vi "cast_meta_idx_toINT.vi"(11 "2D Data Out":sgl[][](array[numeric])) -> (3 "output array":sgl[][](array[numeric]))   [LabVIEW 2017]
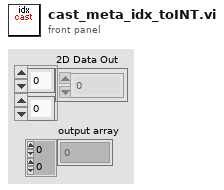
[diagram p1: front panel]
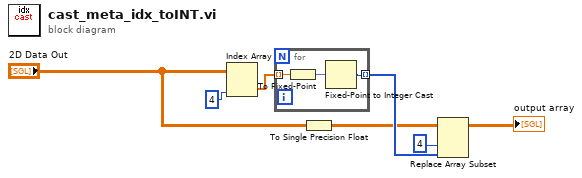
[diagram p0: block diagram]
diagram:
  n1 = Index Array(array="2D Data Out", index (col)=4) -> (element=w6:sgl[])  [unwired: 1 in]
  n2 = for {
    tunnel: w6 -> [w9] mode=indexing
    tunnel: [w10] -> w5 mode=indexing
    n3 = To Fixed-Point(number=w9) -> (fixed-point=w8:fxp<+/-,16,5>)  [unwired: 1 in]
    n4 = Fixed-Point to Integer Cast(1:w8) -> (0:w10:i16)
  }
  n5 = To Single Precision Float(number="2D Data Out") -> (single precision float=w3:sgl[][])
  n6 = Replace Array Subset(array=w3, new element=w5, index (col)=4) -> (→"output array":sgl[][])  [unwired: 1 in]
